vi "Photoresistor.vi"() -> ()   [LabVIEW 2015]
uses:
  <vilib>/Math Plots/2D Math Plots/2D Compass/2D Compass XCtrl/2D Compass.xctl
  <vilib>/DAQmx/read.llb/DAQmx Read (Analog DBL 1Chan 1Samp).vi
  <vilib>/DAQmx/create/channels.llb/DAQmx Create Channel (AI-Voltage-Basic).vi
  <vilib>/DAQmx/miscellaneous.llb/DAQmx Fill In Error Info.vi
  <vilib>/Math Plots/2D Math Plots/2D Compass/2D Compass Datatype/Public/Plot Helper (Complex).vi
  <vilib>/Math Plots/2D Math Plots/2D Compass/2D Compass Datatype/2D Compass Datatype.lvclass
panel:
  in  "stop":bool
  out "error out":errorcluster
  in  "Channel Y":tag="Dev1/ai1"
  in  "Channel X":tag="Dev1/ai0"
  out "2D Compass":refnum<class "2D Plot Datatype.lvclass">[](xcontrol)
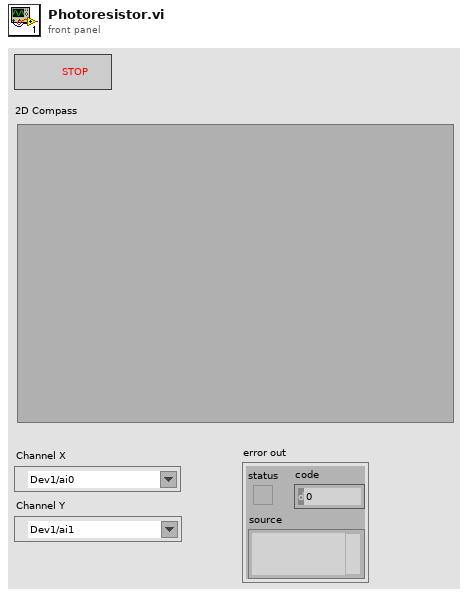
[diagram p1: front panel]
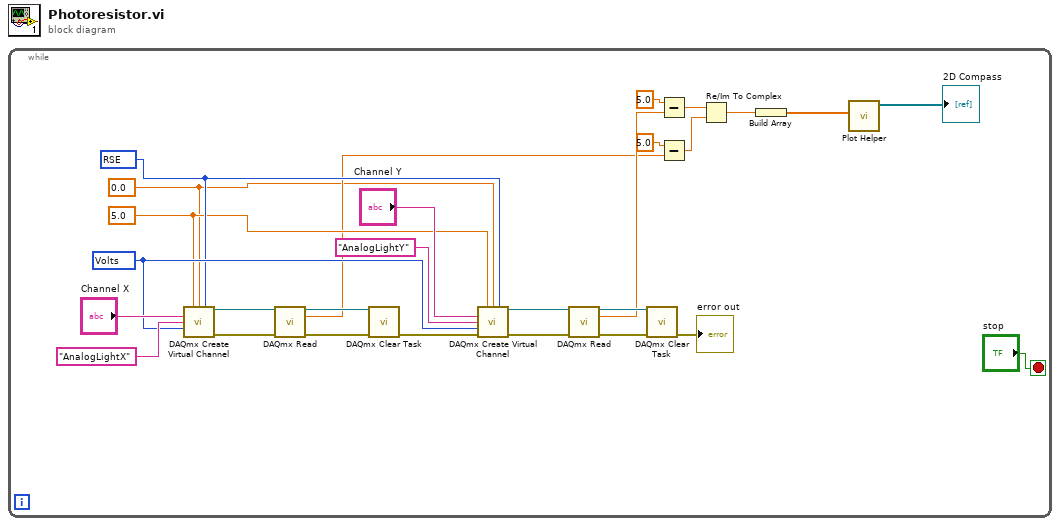
[diagram p0: block diagram]
diagram:
  n1 = while {
    stop <- "stop" stop-if-true
    w21 = 10083 items=["Default"=-1, "RSE"=10083, "NRSE"=10078, "Differential"=10106, "Pseudodifferential"=12529] ("input terminal configuration")
    w1 = 0.0 ("minimum value")
    w20 = 5.0 ("maximum value")
    w22 = 10348 items=["Volts"=10348, "From Custom Scale"=10065] ("units")
    n2 = call-poly <vilib>:"DAQmx Create Virtual Channel.vi"("maximum value"=w20, "minimum value"=w1, "input terminal configuration"=w21, "physical channels"="Channel X", "name to assign"="AnalogLightX" ("Name X"), "units"=w22) -> ("task out"=w16:refnum<k21>, "error out"=w15:errorcluster)  [unwired: 8 in]
    n3 = call-poly <vilib>:"DAQmx Read.vi"("task/channels in"=w16, "error in"=w15) -> ("task out"=w14:refnum<k21>, "data"=w3:dbl, "error out"=w13:errorcluster)  [unwired: 11 in]
    n4 = call <vilib>:"DAQmx Clear Task.vi"("task in"=w14, "error in"=w13) -> ("error out"=w11:errorcluster)  [unwired: 13 in]
    n5 = call-poly <vilib>:"DAQmx Create Virtual Channel.vi"("maximum value"=w20, "minimum value"=w1, "input terminal configuration"=w21, "physical channels"="Channel Y", "name to assign"="AnalogLightY" ("Name Y"), "units"=w22, "error in"=w11) -> ("task out"=w23:refnum<k21>, "error out"=w17:errorcluster)  [unwired: 7 in]
    n6 = call-poly <vilib>:"DAQmx Read.vi"("task/channels in"=w23, "error in"=w17) -> ("task out"=w19:refnum<k21>, "data"=w5:dbl, "error out"=w18:errorcluster)  [unwired: 11 in]
    n7 = call <vilib>:"DAQmx Clear Task.vi"("task in"=w19, "error in"=w18) -> ("error out"=→"error out":errorcluster)  [unwired: 13 in]
    n8 = Subtract(x=5.0, y=w5) -> (x-y=w4:dbl)
    n9 = Subtract(x=5.0, y=w3) -> (x-y=w2:dbl)
    n10 = Re/Im To Complex(1:w2, 2:w4) -> (0:w10:cdb)
    n11 = Build Array(w10) -> (w9:cdb[])
    n12 = call-poly <vilib>:"Plot Helper.vi"("z vector"=w9) -> ("2D Plot Class Obj Array out"=→"2D Compass":refnum<class "2D Plot Datatype.lvclass">[])  [unwired: 2 in, 8 out]
  }
